vi "ConnectFrame.vi"(2 "version":string="1.2") -> (16 "Connect Frame":string)   [LabVIEW 2017, in "LabVIEW STOMP.lvlib" / "STOMP.lvclass"]
uses:
  STOMP.lvclass
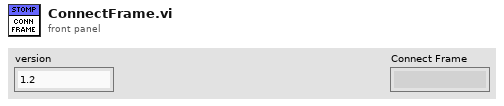
[diagram p1: front panel]
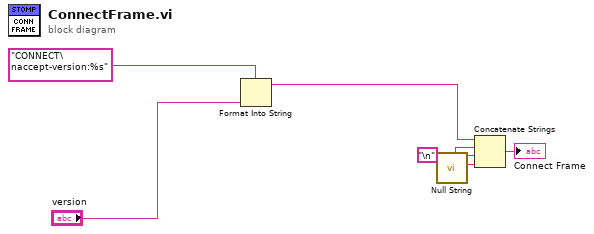
[diagram p0: block diagram]
diagram:
  w6 = "\n"
  n1 = Format Into String(format string="CONNECT\naccept-version:%s" ("address"), "version") -> (resulting string=w2:string)  [unwired: 2 in, 1 out]
  n2 = call "Null String.vi"() -> ("NULL"=w5:string)  [unwired: 19 in]
  n3 = Concatenate Strings(w2, w6, w6, w5) -> (→"Connect Frame":string)
